vi "ScaniValve_client.vi"(0 "Port Number":u8=1 max=47 step=1) -> (1 "Achieved Posn.":T1=8 max=23 step=1, 2 "Diverter Valve":bool, 3 "Error String":string)   [LabVIEW 2014]
uses:
  Anemometry/Anemometry Sub Vis/Baratron Scanning Valve/scanning_valve_tl.ctl
  Sub VIs/ADAM Controls/Update_scan_value.ctl
  Anemometry/Anemometry Sub Vis/Globals/Preference_global.vi
  ADAM Server/Sub VI's/Channel_Description_Global.vi
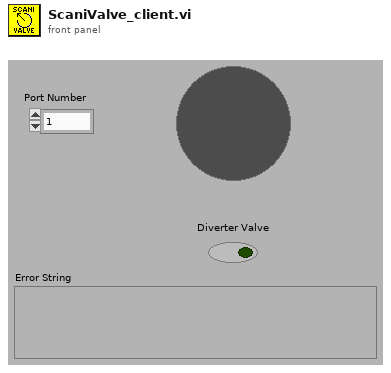
[diagram p1: front panel]
types:
  T1 = typedef "scanning_valve_tl.ctl" = u8
  T2 = typedef "Update_scan_value.ctl" = cluster{"Channel Name":string, "New Value":dbl}
  T3 = enum16{"Load ADAM setup from excel file", "Save ADAM setup to excel file"}
  T4 = typedef "Ch_description_ADAM.ctl" = cluster{"Ch Name":string, "Type":T5, "Function":T6, "Ch State":T7, "Calibration type":T8, "A":dbl, "B":dbl, "C":dbl, "D":dbl, "Comments":string, "Address":T9, "String":string, "Duty":u16}
  T5 = typedef "Module_type_ADAM.ctl" = string
  T6 = typedef "Function_ADAM.ctl" = enum16{"Analogue Input", "Digital Input", "Event counter", "Event rate", "Analogue Output", "Digital Output", "Relay Output"}
  T7 = typedef "Channel_State.ctl" = enum16{"On", "Off", "Always On", "Always Off"}
  T8 = typedef "Calib_type_ADAM.ctl" = enum16{"Raw", "Bx + A", "Cx^2 + Bx + A", "Dx^3 + Cx^2 + Bx + A", "In Band", "Hi-Tec Q", "Hi-Tec M_dot", "Text"}
  T9 = typedef "Address.ctl" = cluster{"Main":i32, "Ch.":i32, "Sub":i32, "Port Name":string}
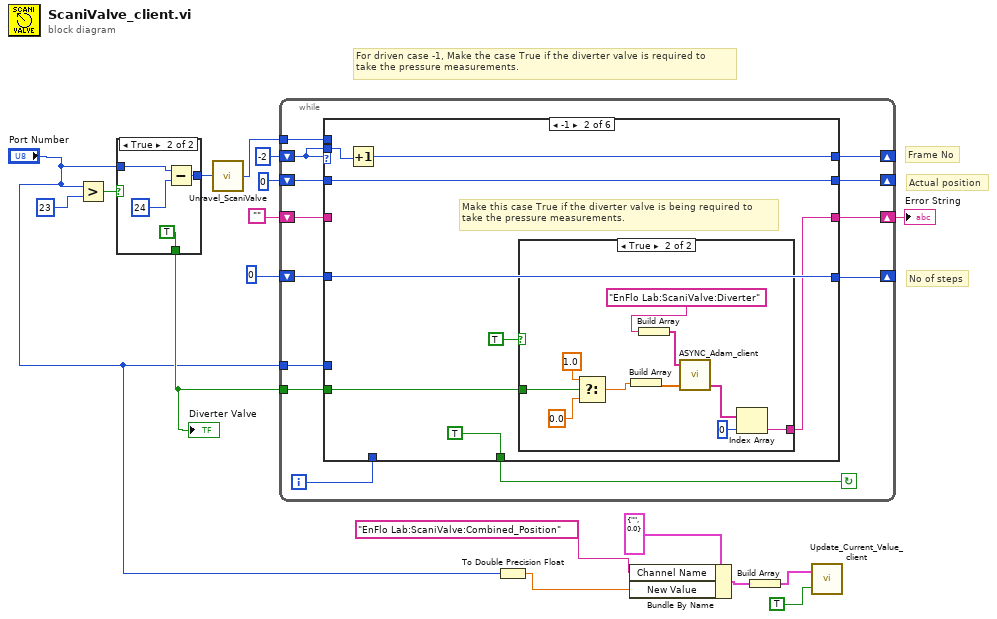
[diagram p0: block diagram]
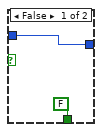
[diagram p2: hidden frame]
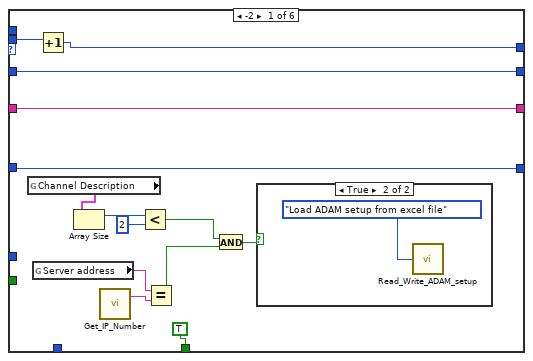
[diagram p3: hidden frame]
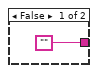
[diagram p5: hidden frame]
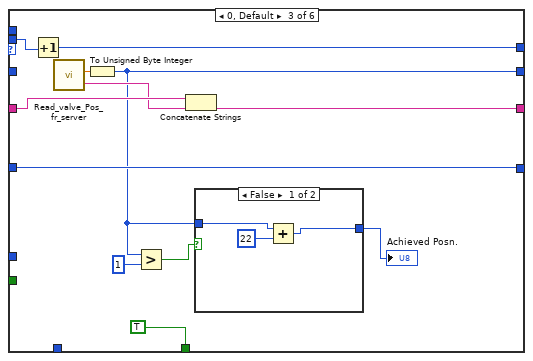
[diagram p6: hidden frame]
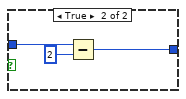
[diagram p7: hidden frame]
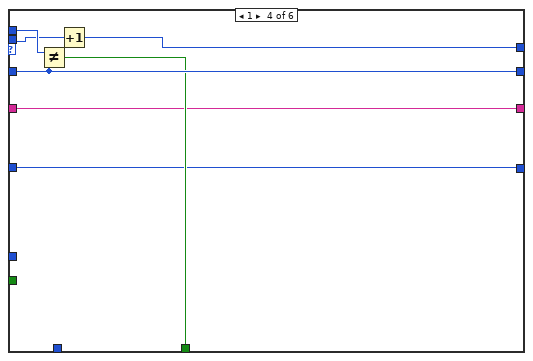
[diagram p8: hidden frame]
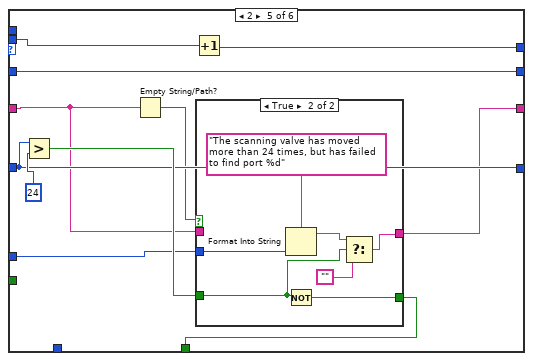
[diagram p9: hidden frame]
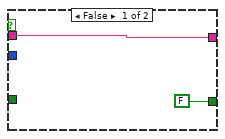
[diagram p10: hidden frame]
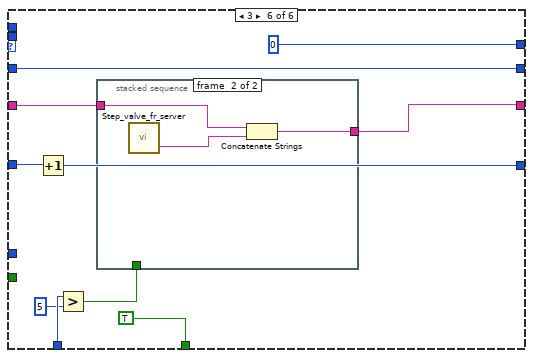
[diagram p11: hidden frame]
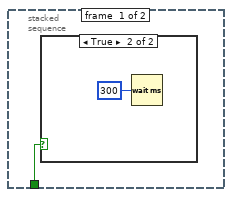
[diagram p12: hidden frame]
diagram:
  # "For driven case -1, Make the case True if the diverter valve is required to \ntake the pressure measurements."
  # "No of steps"
  # "Actual position"
  # "Frame No"
  n1 = Greater?(x="Port Number", y=u8 23) -> (0:w13:bool)
  n2 = case shown="True" w13 {
    tunnel: [FALSE TRUE] -> w12
    tunnel: "Port Number" -> [w18 w22]
    tunnel: [w18 w21] -> w9
    frame False {
    }
    frame True {
      n3 = Subtract(x=w22, y=u8 24) -> (x-y=w21:u8)
    }
  }
  "Diverter Valve" <- w12
  n4 = call "Unravel_ScaniValve.vi"("Port Number"=w9) -> ("Port Number out"=w8:u8)
  n5 = while {
    shift-left: "" -> [w27]
    shift-right: [w28] -> w10
    tunnel: w8 -> [w30]
    shift-left: 0 -> [w32]
    shift-right: [w31] -> _
    shift-left: u8 0 ("Valve Position") -> [w34]
    shift-right: [w35] -> _
    shift-left: -2 -> [w29]
    shift-right: [w36] -> _
    tunnel: w12 -> [w26]
    tunnel: "Port Number" -> [w25]
    i -> [w24]
    stop <- w33 continue-if-true
    n6 = case shown="-1" w29 {
      tunnel: [w49 w59 w82 w91 w103 0] -> w36
      tunnel: [w48 w53 w72 w94 w102 w125] -> w35
      tunnel: w34 -> [w48 w53 _ w94 w102 w125]
      tunnel: w30 -> [_ _ _ w95 _ _]
      tunnel: [TRUE TRUE TRUE w93 w96 TRUE] -> w33
      tunnel: w32 -> [w39 w57 w80 w92 w104 w123]
      tunnel: [w39 w57 w80 w92 w104 w122] -> w31
      tunnel: w29 -> [w50 w56 w78 w90 w101 _]
      tunnel: [w40 w54 w75 w89 w99 w119] -> w28
      tunnel: w27 -> [w40 _ w77 w89 w100 w120]
      tunnel: w26 -> [_ w55 _ _ _ _]
      tunnel: w25 -> [_ _ _ _ w98 _]
      tunnel: w24 -> [_ _ _ _ _ w118]
      frame -2 {
        n7 = global read "Channel_Description_Global.vi" "Channel Description"() -> (w45:T4[])
        n8 = global read "Preference_global.vi" "Server address"() -> (w46:string)
        n9 = Increment(x=w50) -> (x+1=w49:i32)
        n10 = Array Size(array=w45) -> (size(s)=w44:i32)
        n11 = call "Get_IP_Number.vi"() -> ("IP Number"=w47:string)  [unwired: 1 out]
        n12 = Less?(x=w44, y=2) -> (x < y?=w38:bool)
        n13 = Equal?(x=w46, y=w47) -> (x = y?=w42:bool)
        n14 = And(x=w38, y=w42) -> (x .and. y?=w41:bool)
        n15 = case shown="True" w41 {
          frame False {
          }
          frame True {
            n16 = call "Read_Write_ADAM_setup.vi"("Mode"=T3."Load ADAM setup from excel file") -> ()  [unwired: 4 out]
          }
        }
      }
      frame -1 {
        # "Make this case True if the diverter valve is being required to \ntake the pressure measurements."
        n17 = Increment(x=w56) -> (x+1=w59:i32)
        n18 = case shown="True" TRUE {
          tunnel: w55 -> [_ w62]
          tunnel: ["" w61] -> w54
          frame False {
          }
          frame True {
            n19 = Select(t=1.0, s=w62, f=0.0) -> (s? t:f=w65:dbl)
            n20 = Build Array(w65) -> (w66:dbl[])
            n21 = Build Array("EnFlo Lab:ScaniValve:Diverter") -> (w63:string[])
            n22 = call "ASYNC_Adam_client.vi"("Values"=w66, "Channel Names"=w63) -> ("Scan Comments"=w67:string[])  [unwired: 1 in, 1 out]
            n23 = Index Array(array=w67, index=0 ("Index")) -> (element=w61:string)
          }
        }
      }
      frame 0, Default {
        n24 = Increment(x=w78) -> (x+1=w82:i32)
        n25 = call "Read_valve_Pos_fr_server.vi"() -> ("Valve Error Info"=w76:string, "Output Value"=w79:dbl)  [unwired: 1 in, 1 out]
        n26 = To Unsigned Byte Integer(number=w79) -> (unsigned 8bit integer=w72:u8)
        n27 = Greater?(x=w72, y=u8 1) -> (0:w73:bool)
        n28 = Concatenate Strings(w77, w76) -> (w75:string)
        n29 = case shown="False" w73 {
          tunnel: w72 -> [w85 w88]
          tunnel: [w83 w86] -> w71
          frame False {
            n30 = Add(x=w85, y=u8 22) -> (x+y=w83:u8)
          }
          frame True {
            n31 = Subtract(x=w88, y=u8 2) -> (x-y=w86:u8)
          }
        }
        "Achieved Posn." <- w71
      }
      frame 1 {
        n32 = Not Equal?(x=w95, y=w94) -> (x != y?=w93:bool)
        n33 = Increment(x=w90) -> (x+1=w91:i32)
      }
      frame 2 {
        n34 = Greater?(x=w104, y=24) -> (0:w105:bool)
        n35 = Empty String/Path?(string/path=w100) -> (empty?=w97:bool)
        n36 = Increment(x=w101) -> (x+1=w103:i32)
        n37 = case shown="True" w97 {
          tunnel: w105 -> [_ w112]
          tunnel: w100 -> [w108 _]
          tunnel: w98 -> [_ w115]
          tunnel: [w108 w110] -> w99
          tunnel: [FALSE w113] -> w96
          frame False {
          }
          frame True {
            n38 = Format Into String(format string="The scanning valve has moved more than 24 times, but has failed to find port %d" ("Format String"), w115) -> (resulting string=w111:string)  [unwired: 2 in, 1 out]
            n39 = Not(x=w112) -> (.not. x?=w113:bool)
            n40 = Select(t=w111, s=w112, f="") -> (s? t:f=w110:string)
          }
        }
      }
      frame 3 {
        n41 = Increment(x=w123) -> (x+1=w122:i32)
        n42 = Greater?(x=w118, y=5) -> (0:w116:bool)
        n43 = stacked-sequence {
          tunnel: w120 -> [_ w129]
          tunnel: [_ w128] -> w119
          tunnel: w116 -> [w126 _]
          frame #0 {
            n44 = case shown="True" w126 {
              frame False {
              }
              frame True {
                n45 = Wait (ms)(milliseconds to wait=u32 300) -> ()  [unwired: 1 out]
              }
            }
          }
          frame #1 {
            n46 = call "Step_valve_fr_server.vi"() -> ("Valve Error Info"=w130:string)  [unwired: 3 out]
            n47 = Concatenate Strings(w129, w130) -> (w128:string)
          }
        }
      }
    }
  }
  "Error String" <- w10
  n48 = To Double Precision Float(number="Port Number") -> (double precision float=w1:dbl)
  n49 = Bundle By Name(cluster=T2 {"Channel Name"="", "New Value"=0.0} ("Update Scan Value Cluster"), "Channel Name"="EnFlo Lab:ScaniValve:Combined_Position", "New Value"=w1) -> (w5:T2)
  n50 = Build Array(w5) -> (w4:T2[])
  n51 = call "Update_Current_Value_client.vi"("Don't Bother with check?"=TRUE, "Update array in"=w4) -> ()
